vi "GA_Create Population.vi"(5 "Function Data":variant, 6 "Parameters":T1={"Population size"=100, "Generations no."=500, "Significant digits"=4, "Crossover probabality"=0.85, "Mutation mode"=enum."one-point, fixed rate", "Use Gray code?"=FALSE, "Mutation rate"=0.05, "Min mutation rate"=0.0005, "Max mutation rate"=0.25, "Reproduction plan"=enum."Steady-state-replace-worst", "Elitism"=FALSE, "Fmax"=1} {"Max mutation rate" min=0.0 max=1.0; "Min mutation rate" min=0.0 max=1.0; "Mutation rate" min=0.0 max=1.0; "Crossover probabality" min=0.0 max=1.0; "Significant digits" min=1; "Generations no." min=1; "Population size" min=1}, 7 "Fitness Function":T3, 8 "Phenotype size":i32, 9 "Population size":i32) -> (3 "Population out":T2)   [LabVIEW 2016, in "Optimal Frequency Bands Search.lvlib" / "GeneticAlgorithm.lvlib"]
doc: "Случайным образом создать особей для начальной популяции"
uses:
  GeneticAlgorithm.lvlib
  GA_tFitness Function.ctl
  GA_tPopulation.ctl
  GA_tParameters.ctl
  <vilib>/gmath/statdist.llb/Uniform (Discrete) Random.vi
  <vilib>/gmath/NI_Gmath.lvlib
  particle_swarm_opt/ParticleSwarm.lvlib
panel:
  # "This VI is a part of BCI Design library, http://www.ru-bci.org \nCopyright © 2020, Sotnikov Peter, All rights reserved. License: CC BY-NC 4.0"
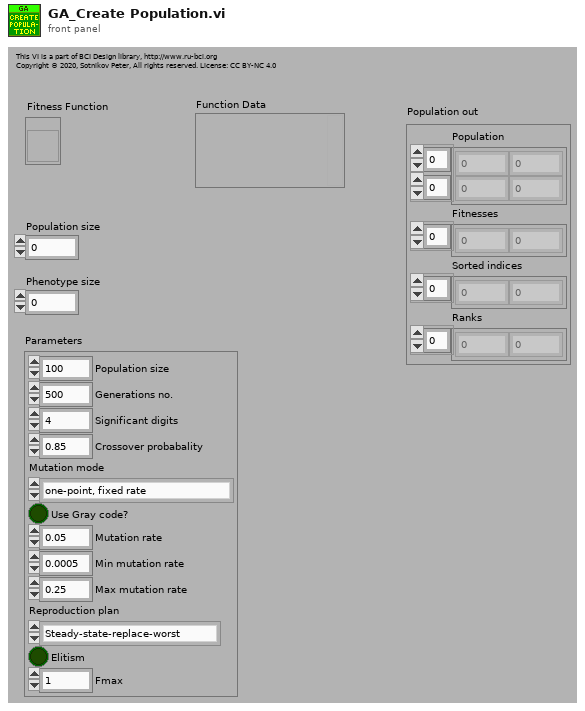
[diagram p1: front panel]
types:
  T1 = typedef "Optimal Frequency Bands Search.lvlib/GeneticAlgorithm.lvlib/GA_tParameters.ctl" = cluster{"Population size":i32, "Generations no.":i32, "Significant digits":i32, "Crossover probabality":dbl, "Mutation mode":enum16{"one-point, fixed rate", "one-point, fitness-adjustable rate", "one-point, distance-adjustable rate"}, "Use Gray code?":bool, "Mutation rate":dbl, "Min mutation rate":dbl, "Max mutation rate":dbl, "Reproduction plan":enum16{"Full generational replacement", "Steady-state-replace-random", "Steady-state-replace-worst"}, "Elitism":bool, "Fmax":i32}
  T2 = typedef "Optimal Frequency Bands Search.lvlib/GeneticAlgorithm.lvlib/GA_tPopulation.ctl" = cluster{"Population":i32[][], "Fitnesses":dbl[], "Sorted indices":i32[], "Ranks":i32[]}
  T3 = typedef "Optimal Frequency Bands Search.lvlib/GeneticAlgorithm.lvlib/GA_tFitness Function.ctl" = refnum<vi>
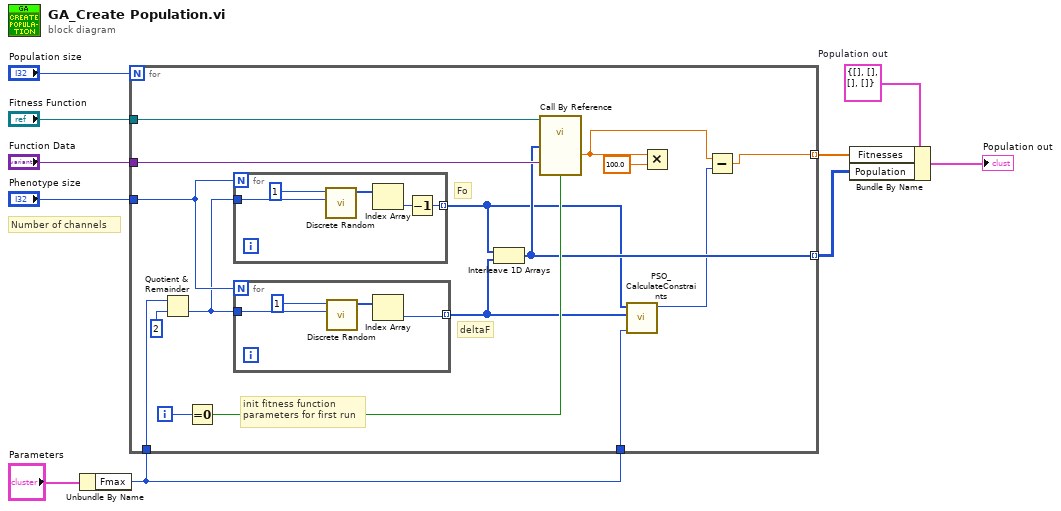
[diagram p0: block diagram]
diagram:
  w7 = T2 {"Population"=[], "Fitnesses"=[], "Sorted indices"=[], "Ranks"=[]}  # Population out
  # "Number of channels"
  n1 = Unbundle By Name("Parameters") -> ("Fmax"=w1:i32)
  n2 = for {
    N: "Population size" -> [_]
    tunnel: "Phenotype size" -> [w21]
    tunnel: "Fitness Function" -> [w25]
    tunnel: [w15] -> w6 mode=indexing
    tunnel: [w22] -> w5 mode=indexing
    tunnel: "Function Data" -> [w26]
    tunnel: w1 -> [w18]
    tunnel: w1 -> [w14]
    i -> [w24]
    # "deltaF"
    # "Fo"
    # "init fitness function\nparameters for first run"
    n3 = Quotient & Remainder(x=w14, y=2) -> (floor(x/y)=w12:i32)  [unwired: 1 out]
    n4 = Equal To 0?(x=w24) -> (x = 0?=w23:bool)
    n5 = for {
      N: w21 -> [_]
      tunnel: [w32] -> w20 mode=indexing
      tunnel: w12 -> [w31]
      n6 = call-poly <vilib>:"Discrete Random.vi"("n"=w31, "samples"=1) -> ("uniform (discrete) random data"=w34:i32[])  [unwired: 8 in, 1 out]
      n7 = Index Array(array=w34) -> (element=w33:i32)  [unwired: 1 in]
      n8 = Decrement(x=w33) -> (x-1=w32:i32)
    }
    n9 = for {
      N: w21 -> [_]
      tunnel: [w28] -> w19 mode=indexing
      tunnel: w12 -> [w27]
      n10 = call-poly <vilib>:"Discrete Random.vi"("n"=w27, "samples"=1) -> ("uniform (discrete) random data"=w29:i32[])  [unwired: 8 in, 1 out]
      n11 = Index Array(array=w29) -> (element=w28:i32)  [unwired: 1 in]
    }
    n12 = Interleave 1D Arrays(w20, w19) -> (w22:i32[])
    n13 = call-by-ref "Call By Reference"(reference=w25, "Init? (F)"=w23, "Data"=w26, "Phenotype"=w22) -> ("Fitness"=w11:dbl)  [unwired: 1 in, 2 out]
    n14 = call "PSO_CalculateConstraints.vi"("Fmax"=w18, "deltaF vector"=w19, "F0 vector"=w20) -> ("Penalty"=w16:i32)  [unwired: 7 in, 1 out]
    n15 = Multiply(x=w11, y=100.0) -> ()  [unwired: 1 out]
    n16 = Subtract(x=w11, y=w16) -> (x-y=w15:dbl)
  }
  n17 = Bundle By Name(cluster=w7, "Fitnesses"=w6, "Population"=w5) -> (→"Population out":T2)
